vi "Configure Harmonics Characteristics.vi"(4 "Select Order (0: All)":i32(ring) items=["All", "Even", "Odd"], 6 "Max Order (0: All)":i32 min=0 max=500, 7 "Item (1)":i32=1 min=1 max=64 step=1, 8 "error in (no error)":errorcluster, 9 "Element/Wiring Unit (1: 1)":i32(ring)=1 items=["1"=1, "2"=2, "3"=3, "4"=4, "5"=5, "6"=6, "Sigma A"=7, "Sigma B"=8, "Sigma C"=9], 10 "Function (0: None)":i32(ring) items=["None", "U", "I", "P", "S", "Q", "Lambda", "Phi", "Phi U", "Phi I", "Z", "Rs", "Xs", "Rp", "Xp", "UHDF", "IHDF", "PHDF"], 11 "VISA resource name":refnum<visa-resource-name>) -> (0 "error out":errorcluster, 3 "VISA resource name out":refnum<visa-resource-name>)   [LabVIEW 2021, in "Yokogawa WT1800 Series.lvlib"]
doc: "Configures the harmonics numeric features.\n\n<b>Note:</b>\nThis setting valid on models with the harmonic\nmeasurement (/G5 or /G6) option."
uses:
  <instrlib>/Yokogawa WT1800 Series/Yokogawa WT1800 Series.lvlib
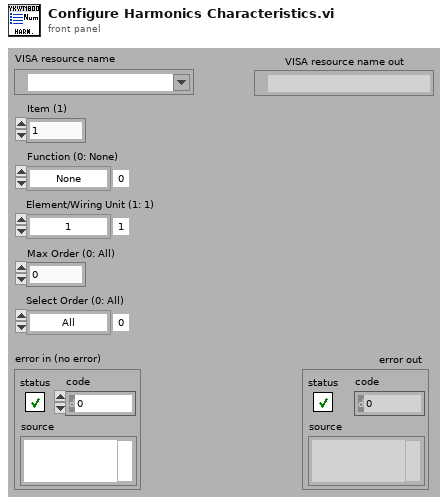
[diagram p1: front panel]
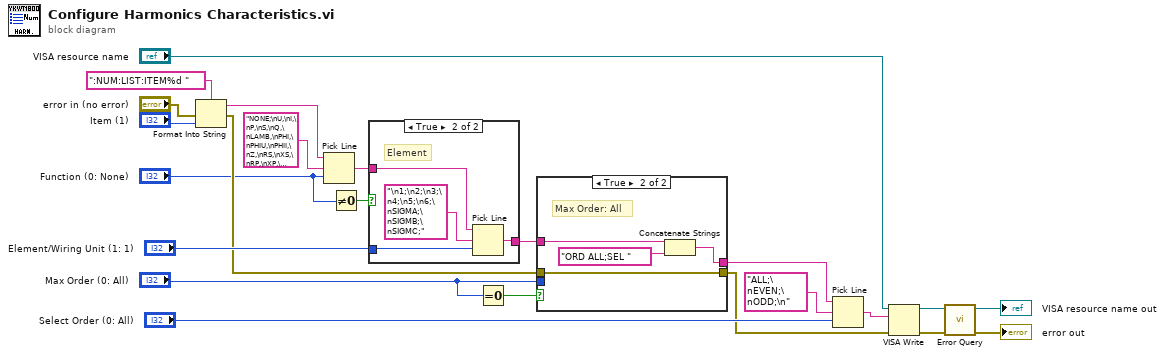
[diagram p0: block diagram]
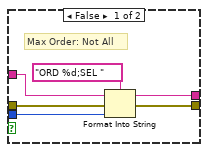
[diagram p3: hidden frame]
diagram:
  n1 = Format Into String(format string=":NUM:LIST:ITEM%d " ("形式文字列"), error in="error in (no error)", "Item (1)") -> (resulting string=w14:string, error out=w8:errorcluster)  [unwired: 1 in]
  n2 = Pick Line ("ライン選択")(string ("")=w14, multi-line string="NONE;\nU,\nI,\nP,\nS,\nQ,\nLAMB,\nPHI,\nPHIU,\nPHII,\nZ,\nRS,\nXS,\nRP,\nXP,\nUHDF,\nIHDF,\nPHDF," ("複数行文字列"), line index="Function (0: None)") -> (output string=w13:string)
  n3 = Not Equal To 0?(x="Function (0: None)") -> (x != 0?=w2:bool)
  n4 = case shown="True" w2 {
    tunnel: w13 -> [w24 w27]
    tunnel: "Element/Wiring Unit (1: 1)" -> [_ w26]
    tunnel: [w24 w25] -> w9
    frame False {
      # "Function: None"
    }
    frame True {
      # "Element"
      n5 = Pick Line ("ライン選択")(string ("")=w27, multi-line string="\n1;\n2;\n3;\n4;\n5;\n6;\nSIGMA;\nSIGMB;\nSIGMC;" ("複数行文字列"), line index=w26) -> (output string=w25:string)
    }
  }
  n6 = Equal To 0?(x="Max Order (0: All)") -> (x = 0?=w11:bool)
  n7 = case shown="True" w11 {
    tunnel: "Max Order (0: All)" -> [w33 _]
    tunnel: w9 -> [w32 w37]
    tunnel: w8 -> [w31 w35]
    tunnel: [w30 w36] -> w6
    tunnel: [w29 w35] -> w3
    frame False {
      # "Max Order: Not All"
      n8 = Format Into String(format string="ORD %d;SEL " ("形式文字列"), initial string=w32, error in=w31, w33) -> (resulting string=w30:string, error out=w29:errorcluster)
    }
    frame True {
      # "Max Order: All"
      n9 = Concatenate Strings(w37, "ORD ALL;SEL " ("文字列")) -> (w36:string)
    }
  }
  n10 = Pick Line ("ライン選択")(string ("")=w6, multi-line string="ALL;\nEVEN;\nODD;\n" ("複数行文字列"), line index="Select Order (0: All)") -> (output string=w4:string)
  n11 = VISA Write ("VISA書き込み")(VISA resource name="VISA resource name", write buffer=w4, error in (no error)=w3) -> (VISA resource name out=w23:refnum<visa-resource-name>, error out=w22:errorcluster)  [unwired: 1 out]
  n12 = call <instrlib>:"Error Query.vi"("error in (no error)"=w22, "VISA resource name"=w23) -> ("error out"=→"error out":errorcluster, "VISA resource name out"=→"VISA resource name out":refnum<visa-resource-name>)  [unwired: 6 in, 2 out]
